vi "test_CCDRestart.vi"(8 "error in":errorcluster, 9 "tear down connection":bool=TRUE) -> (0 "error out":errorcluster)   [LabVIEW 2023]
uses:
  <vilib>/addons/_JKI Toolkits/Caraya/classes/Test/Test.lvclass
  <vilib>/addons/_JKI Toolkits/Caraya/classes/Assert/Assert.lvclass
  horiba.test.lvlib
  <vilib>/addons/_JKI Toolkits/Caraya/classes/Assert/Assert Not Error.vi
  Classes/CCD/CCD.lvclass
  <vilib>/addons/_JKI Toolkits/Caraya/classes/Assert/Assert Error.vi
  Classes/GenericDevice/GenericDevice.lvclass
panel:
  # "Connector Pane"
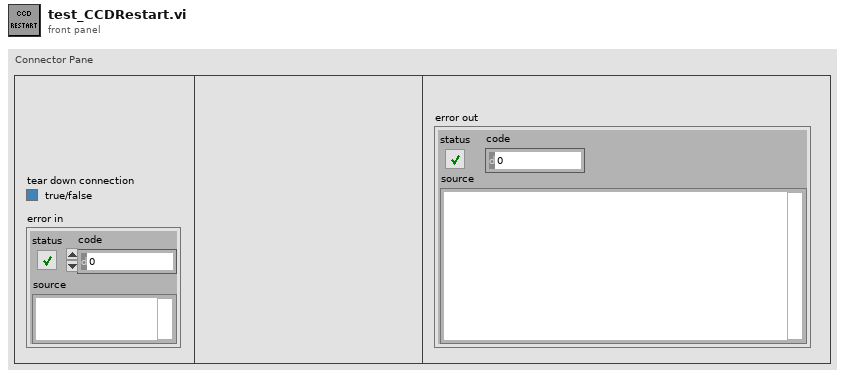
[diagram p1: front panel]
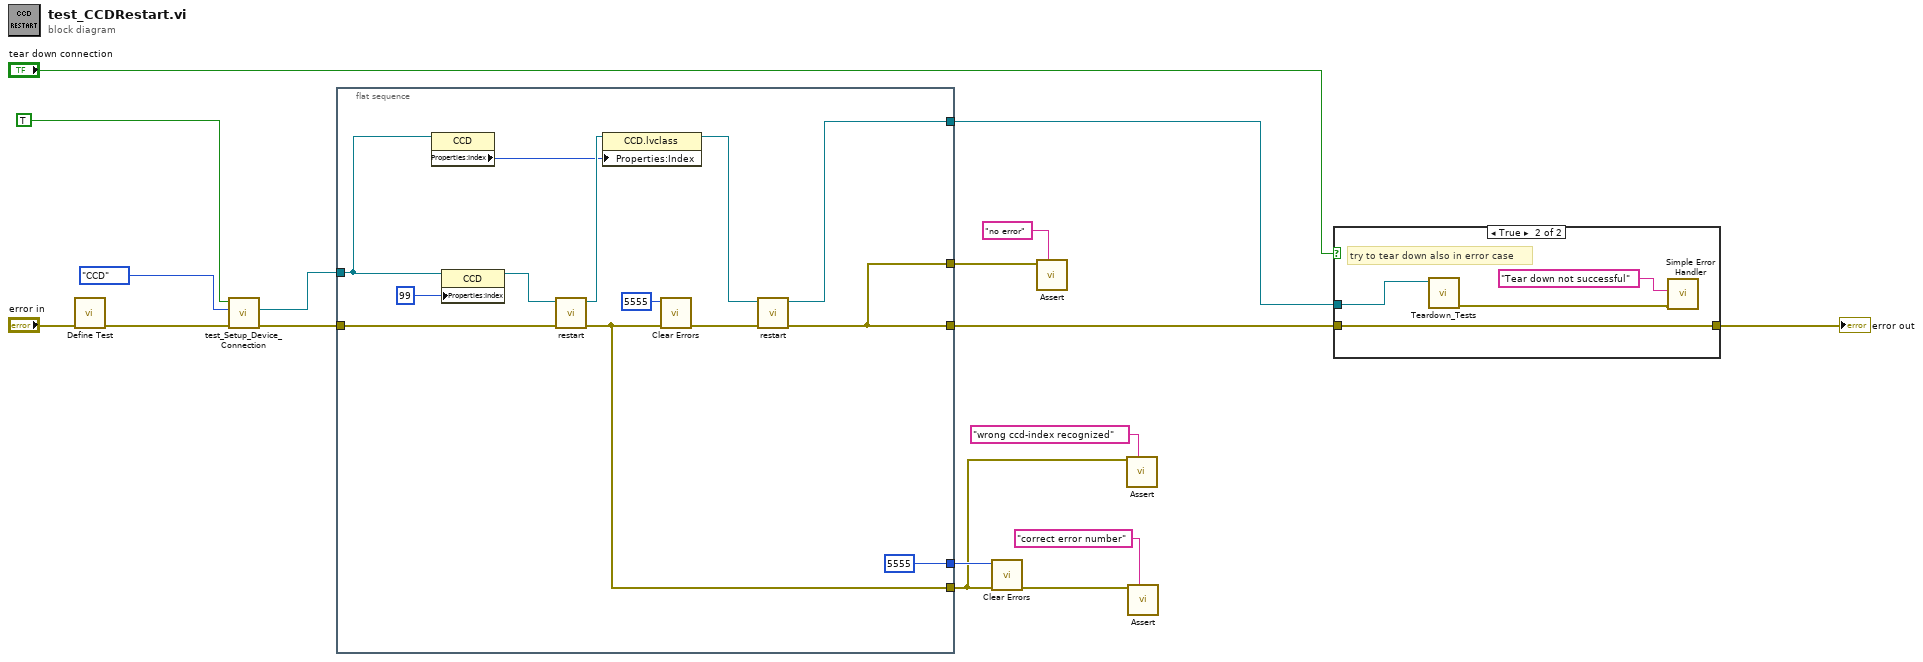
[diagram p0: block diagram]
diagram:
  n1 = call <vilib>:"Define Test.vi"("error in (no error)"="error in") -> ("error out"=w10:errorcluster)  [unwired: 9 in, 1 out]
  n2 = call "test_Setup_Device_Connection.vi"("error in (no error)"=w10, "device selection"=enum16{"monochromator", "CCD", "SCD"}."CCD", "set-up a connection"=TRUE) -> ("error out"=w8:errorcluster, "CCD out"=w9:refnum<class "CCD.lvclass">)  [unwired: 5 in, 2 out]
  n3 = flat-sequence {
    tunnel: w8 -> [w30]
    tunnel: w9 -> [w29]
    tunnel: [w21] -> w4
    tunnel: [w23] -> w13
    tunnel: [5555] -> w7
    tunnel: [w18] -> w3
    tunnel: [w18] -> w1
    frame #0 {
      n4 = property class="CCD"(reference=w29) -> ("Properties:Index"=w25:i32)  [unwired: 1 in, 2 out]
      n5 = property class="CCD"(reference=w29, "Properties:Index"=99 ("Index")) -> (reference out=w28:refnum<class "CCD.lvclass">)  [unwired: 1 in, 1 out]
      n6 = call "restart.vi"("error in (no error)"=w30, "CCD in"=w28) -> ("error out"=w21:errorcluster, "CCD out"=w26:refnum<class "CCD.lvclass">)  [unwired: 6 in, 2 out]
      n7 = property class="CCD.lvclass"(reference=w26, "Properties:Index"=w25) -> (reference out=w24:refnum<class "CCD.lvclass">)  [unwired: 1 in, 1 out]
      n8 = call <vilib>:"Clear Errors.vi"("error in (no error)"=w21, "specific error code to clear (0: all)"=5555) -> ("error out"=w20:errorcluster)  [unwired: 4 in, 1 out]
      n9 = call "restart.vi"("error in (no error)"=w20, "CCD in"=w24) -> ("error out"=w18:errorcluster, "CCD out"=w23:refnum<class "CCD.lvclass">)  [unwired: 6 in, 2 out]
    }
  }
  n10 = call <vilib>:"Clear Errors.vi"("error in (no error)"=w4, "specific error code to clear (0: all)"=w7) -> ("error out"=w6:errorcluster)  [unwired: 4 in, 1 out]
  n11 = call-poly <vilib>:"Assert.vi"("Label"="no error" ("Label (VI Title)"), "Not Error?"=w3) -> ()  [unwired: 8 in, 2 out]
  n12 = call-poly <vilib>:"Assert.vi"("Label"="wrong ccd-index recognized" ("Label (VI Title)"), "Error?"=w4) -> ()  [unwired: 8 in, 2 out]
  n13 = call-poly <vilib>:"Assert.vi"("Label"="correct error number" ("Label (VI Title)"), "Not Error?"=w6) -> ()  [unwired: 8 in, 2 out]
  n14 = case shown="True" "tear down connection" {
    tunnel: w13 -> [_ w34]
    tunnel: [w31 w32] -> w2
    tunnel: w1 -> [w31 w32]
    frame False {
    }
    frame True {
      # "try to tear down also in error case"
      n15 = call "Teardown_Tests.vi"("horiba.lvlib:GenericDevice"=w34) -> ("error out"=w33:errorcluster)  [unwired: 9 in, 1 out]
      n16 = call <vilib>:"Simple Error Handler.vi"("error source (\" \")"="Tear down not successful" ("error source (\" \")"), "error in (no error)"=w33) -> ()  [unwired: 3 in, 5 out]
    }
  }
  "error out" <- w2
